vi "Read N.vi"(8 "error in (no error)":errorcluster, 11 "MB_TCP in":refnum<class "MB_TCP.lvclass">) -> (0 "error out":errorcluster, 2 "N":i32, 3 "MB_TCP out":refnum<class "MB_TCP.lvclass">)   [LabVIEW 2021, in "MB_TCP.lvclass"]
uses:
  MB_TCP.lvclass
  MB_TCP.lvclass/MB_TCP.ctl
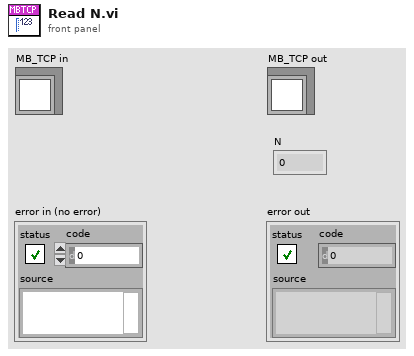
[diagram p1: front panel]
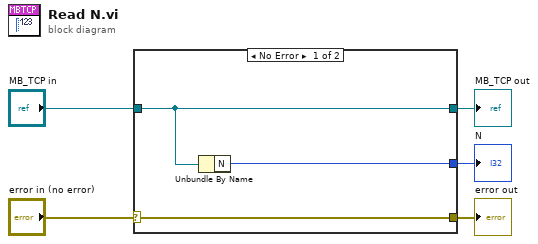
[diagram p0: block diagram]
diagram:
  n1 = case shown="No Error" "error in (no error)" {
    selector: "error in (no error)" -> [w8 w10]
    tunnel: [w8 w10] -> w4
    tunnel: [w6 w9] -> w1
    tunnel: "MB_TCP in" -> [w6 w9]
    tunnel: [w7 _] -> w3
    frame No Error {
      n2 = Unbundle By Name(w6) -> ("N"=w7:i32)
    }
    frame Error {
    }
  }
  "error out" <- w4
  "N" <- w3
  "MB_TCP out" <- w1
